vi "C2D_ZPK_bilinearTransform.vi"(8 "error in (no error)":errorcluster, 10 "Sampling Time (Ts) [s]":dbl, 11 "ZPK model (CT)":T1) -> (0 "error out":errorcluster, 3 "ZPK model (DT)":T1)   [LabVIEW 2020, in "PC-RT_Controller.lvlib"]
doc: "Convert continuous time zero-pole-gain (ZPK) model into discrete ZPK model using bilinear (tustin) transform."
uses:
  PC-RT_Controller.lvlib
  TypeDefs/ZPK_model.ctl
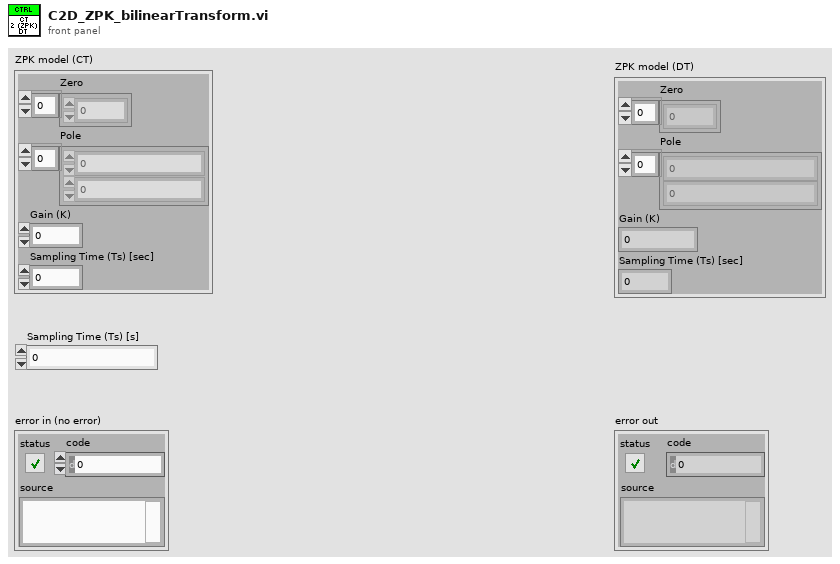
[diagram p1: front panel]
types:
  T1 = typedef "PC-RT_Controller.lvlib/ZPK_model.ctl" = cluster{"Zero":cdb[], "Pole":cdb[], "Gain (K)":dbl, "Sampling Time (Ts) [sec]":dbl}
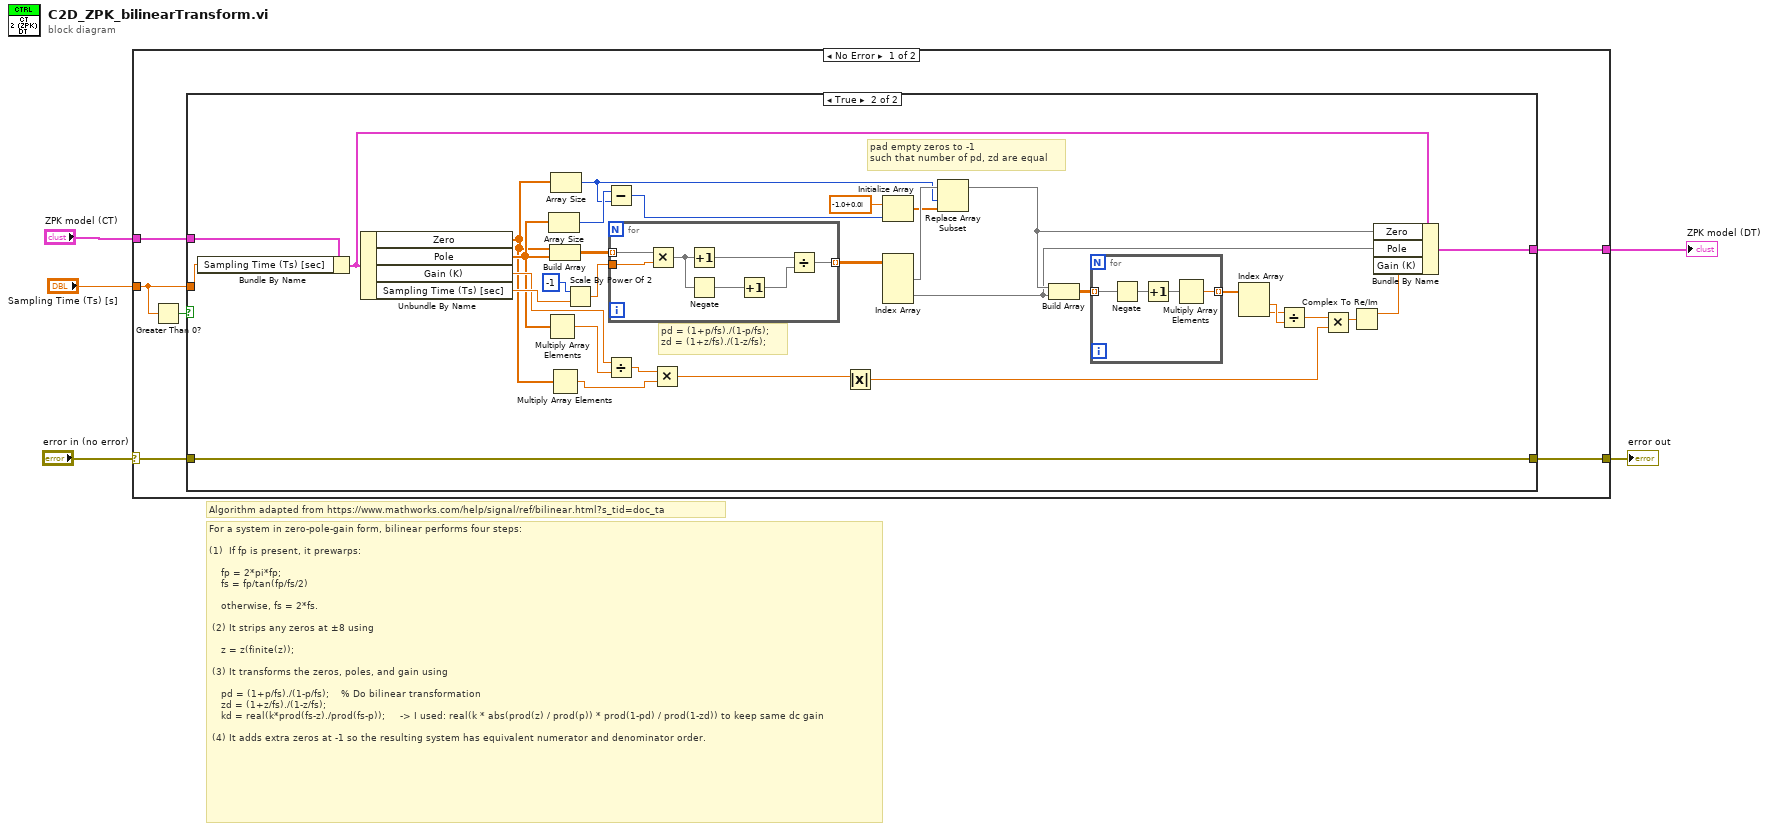
[diagram p0: block diagram]
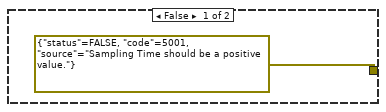
[diagram p2: hidden frame]
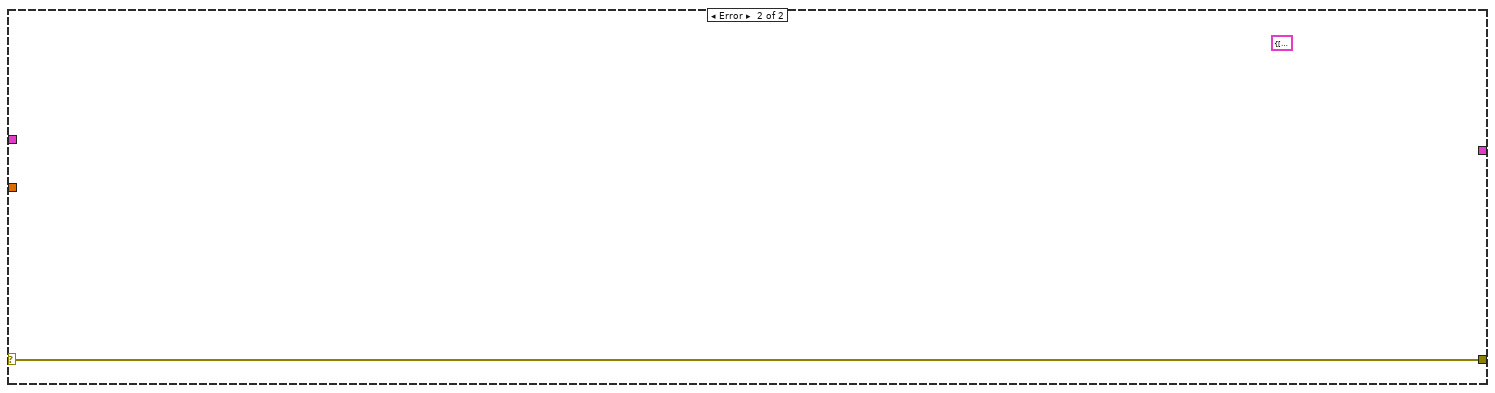
[diagram p3: hidden frame]
diagram:
  # "For a system in zero-pole-gain form, bilinear performs four steps:\n\n(1)  If fp is present, it prewarps:\n\n    fp = 2*pi*fp;\n    fs = fp/tan(fp/fs/2)\n\n    otherwise, fs = 2*fs.\n\n (2) It strips any zeros at ±8 using\n\n    z = z(finite(z));\n\n (3) It transforms the zeros, poles, and gain using\n\n    pd = (1+p/fs)./(1-p/fs);    % Do bilinear transformation\n    zd = (1+z/fs)./(1-z/fs);\n    kd = real(k*prod(fs-z)./prod(fs-p));     -> I used: real(k * abs(prod(z) / prod(p)) * prod(1-pd) / prod(1-zd)) to keep same dc gain\n\n (4) It adds extra zeros at -1 so the resulting system has equivalent numerator and denominator order."
  # "Algorithm adapted from https://www.mathworks.com/help/signal/ref/bilinear.html?s_tid=doc_ta"
  n1 = case shown="No Error" "error in (no error)" {
    selector: "error in (no error)" -> [w7 w57]
    tunnel: "ZPK model (CT)" -> [w11 _]
    tunnel: [w6 w57] -> w4
    tunnel: "Sampling Time (Ts) [s]" -> [w8 _]
    tunnel: [w10 _] -> w1
    frame No Error {
      n2 = Greater Than 0?(x=w8) -> (x > 0?=w9:bool)
      n3 = case shown="True" w9 {
        tunnel: w11 -> [_ w45]
        tunnel: w8 -> [_ w44]
        tunnel: [_ w24] -> w10
        tunnel: w7 -> [_ w15]
        tunnel: [errorcluster {"status"=FALSE, "code"=5001, "source"="Sampling Time should be a positive value."} ("error IO") w15] -> w6
        frame False {
        }
        frame True {
          # "pad empty zeros to -1 \nsuch that number of pd, zd are equal"
          # "pd = (1+p/fs)./(1-p/fs); \nzd = (1+z/fs)./(1-z/fs);"
          n4 = Bundle By Name(cluster=w45, "Sampling Time (Ts) [sec]"=w44) -> (w16:T1)
          n5 = Unbundle By Name(w16) -> ("Zero"=w21:cdb[], "Pole"=w29:cdb[], "Gain (K)"=w31:dbl, "Sampling Time (Ts) [sec]"=w42:dbl)
          n6 = Multiply Array Elements(1:w29) -> (0:w30:cdb)
          n7 = Array Size(array=w29) -> (size(s)=w39:i32)
          n8 = Build Array(w21, w29) -> (w40:cdb[][])
          n9 = Multiply Array Elements(1:w21) -> (0:w19:cdb)
          n10 = Array Size(array=w21) -> (size(s)=w35:i32)
          n11 = Scale By Power Of 2(n=i16 -1, x=w42) -> (x*2^n=w33:dbl)
          n12 = Subtract(x=w39, y=w35) -> (x-y=w38:i32)
          n13 = Divide(x=w31, y=w30) -> (x/y=w20:cdb)
          n14 = for {
            tunnel: w40 -> [w52] mode=indexing
            tunnel: w33 -> [w51]
            tunnel: [w50] -> w41 mode=indexing
            n15 = Multiply(x=w52, y=w51) -> (x*y=w49:cdb[])
            n16 = Increment(x=w49) -> (x+1=w47:cdb[])
            n17 = Negate(x=w49) -> (-x=w48:cdb[])
            n18 = Increment(x=w48) -> (x+1=w46:cdb[])
            n19 = Divide(x=w47, y=w46) -> (x/y=w50:cdb[])
          }
          n20 = Multiply(x=w20, y=w19) -> (x*y=w14:cdb)
          n21 = Absolute Value(x=w14) -> (abs(x)=w13:dbl)
          n22 = Initialize Array(cdb -1.0+0.0i ("element"), w38) -> (w34:cdb[])
          n23 = Index Array(array=w41) -> (element #1=w36:cdb[], element #2=w22:cdb[])  [unwired: 4 in]
          n24 = Replace Array Subset(array=w36, new element=w34, index=w35) -> (w23:cdb[])
          n25 = Build Array(w23, w22) -> (w32:cdb[][])
          n26 = for {
            tunnel: w32 -> [w53] mode=indexing
            tunnel: [w54] -> w28 mode=indexing
            n27 = Negate(x=w53) -> (-x=w56:cdb[])
            n28 = Increment(x=w56) -> (x+1=w55:cdb[])
            n29 = Multiply Array Elements(1:w55) -> (0:w54:cdb)
          }
          n30 = Index Array(array=w28) -> (element #1=w27:cdb, element #2=w26:cdb)  [unwired: 2 in]
          n31 = Divide(x=w26, y=w27) -> (x/y=w25:cdb)
          n32 = Multiply(x=w25, y=w13) -> (x*y=w18:cdb)
          n33 = Complex To Re/Im(x + iy=w18) -> (x=w17:dbl)  [unwired: 1 out]
          n34 = Bundle By Name(cluster=w16, "Zero"=w23, "Pole"=w22, "Gain (K)"=w17) -> (w24:T1)
        }
      }
    }
    frame Error {
      (unwired) cluster{"Zero":cdb[], "Pole":cdb[], "Gain":dbl} {"Zero"=[], "Pole"=[], "Gain"=0.0} ("ZPK (polar form)")
    }
  }
  "ZPK model (DT)" <- w1
  "error out" <- w4
